vi "Realsense Cam Stream Profile Convert.vi"(8 "error in (no error)":errorcluster, 10 "Numeric":i32, 11 "Profiles_list_out":u64) -> (0 "error out":errorcluster, 3 "output cluster":T1={"ID"=2, "Profile"=357735784, "fps"=25, "RS Stream"=3, "RS Format"=10, "index"=2, "width"=1920, "height"=1080, "ppx"=0.0, "ppy"=0.0, "fx"=0.0, "fy"=0.0, "model"=0} {"model" items=["RS_DISTORTION_NONE"=0, "RS_DISTORTION_MODIFIED_BROWN_CONRADY"=1, "RS_DISTORTION_INVERSE_BROWN_CONRADY"=2, "RS_DISTORTION_COUNT"=3, "RS_DISTORTION_MAX_ENUM"=2147483647]})   [LabVIEW 2018, in "Realsense Cam.lvclass"]
uses:
  Realsense Cam.lvclass
  realsense_wrapper_api/libRealSense3.lvlib
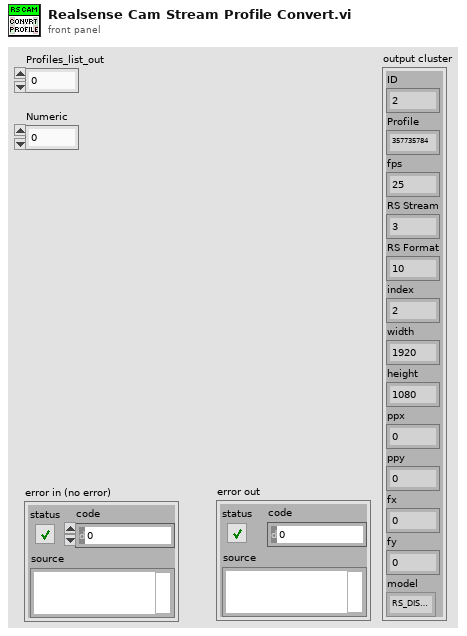
[diagram p1: front panel]
types:
  T1 = cluster{"ID":i32, "Profile":u64, "fps":i32, "RS Stream":u16, "RS Format":u16, "index":u16, "width":u16, "height":u16, "ppx":sgl, "ppy":sgl, "fx":sgl, "fy":sgl, "model":u32}
  T2 = cluster{"width":i32, "height":i32, "ppx":sgl, "ppy":sgl, "fx":sgl, "fy":sgl, "model":u32, "coeffs[0]":sgl, "coeffs[1]":sgl, "coeffs[2]":sgl, "coeffs[3]":sgl, "coeffs[4]":sgl}
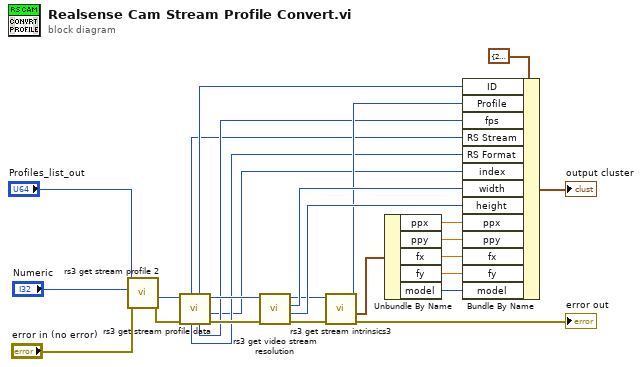
[diagram p0: block diagram]
diagram:
  n1 = call "rs3 get stream profile 2.vi"("error in (no error)"="error in (no error)", "index"="Numeric", "Stream Profile list in"="Profiles_list_out") -> ("error out"=w22:errorcluster, "stream profile"=w21:u64)  [unwired: 5 in, 2 out]
  n2 = call "rs3 get stream profile data.vi"("error in (no error)"=w22, "Profile"=w21) -> ("error out"=w24:errorcluster, "index"=w2:i32, "Profile out"=w23:u64, "frame rate"=w5:i32, "unique id"=w8:i32, "RS Format"=w3:u16, "RS Stream"=w4:u16)  [unwired: 2 in, 1 out]
  n3 = call "rs3 get video stream resolution.vi"("error in (no error)"=w24, "Profile"=w23) -> ("error out"=w25:errorcluster, "height"=w9:u32, "width"=w10:u32, "Profile out"=w7:u64)  [unwired: 5 in, 1 out]
  n4 = call "rs3 get stream intrinsics3.vi"("error in (no error)"=w25, "stream profile"=w7) -> ("error out"=→"error out":errorcluster, "intrin out"=w16:T2, "stream profile out"=w6:u64)  [unwired: 6 in, 1 out]
  n5 = Unbundle By Name(w16) -> ("ppx"=w15:sgl, "ppy"=w14:sgl, "fx"=w13:sgl, "fy"=w12:sgl, "model"=w11:u32)
  n6 = Bundle By Name(cluster=T1 {"ID"=2, "Profile"=357735784, "fps"=25, "RS Stream"=3, "RS Format"=10, "index"=2, "width"=1920, "height"=1080, "ppx"=0.0, "ppy"=0.0, "fx"=0.0, "fy"=0.0, "model"=0} ("output cluster 2"), "ID"=w8, "Profile"=w6, "fps"=w5, "RS Stream"=w4, "RS Format"=w3, "index"=w2, "width"=w10, "height"=w9, "ppx"=w15, "ppy"=w14, "fx"=w13, "fy"=w12, "model"=w11) -> (→"output cluster":T1)
